vi "Gas Ritter Temperature and Pressure.vi"(0 "Ritter Data":T1, 5 "TC8":dbl, 7 "PSI 1":dbl, 9 "Heise Barometric Pressure (inHG)":dbl, 11 "error in (no error)":errorcluster) -> (4 "Ritter Data Output":T1, 15 "error out":errorcluster)   [LabVIEW 2023]
uses:
  Drivers/Ritter Gas Meter/Type Definitions/Ritter Data.ctl
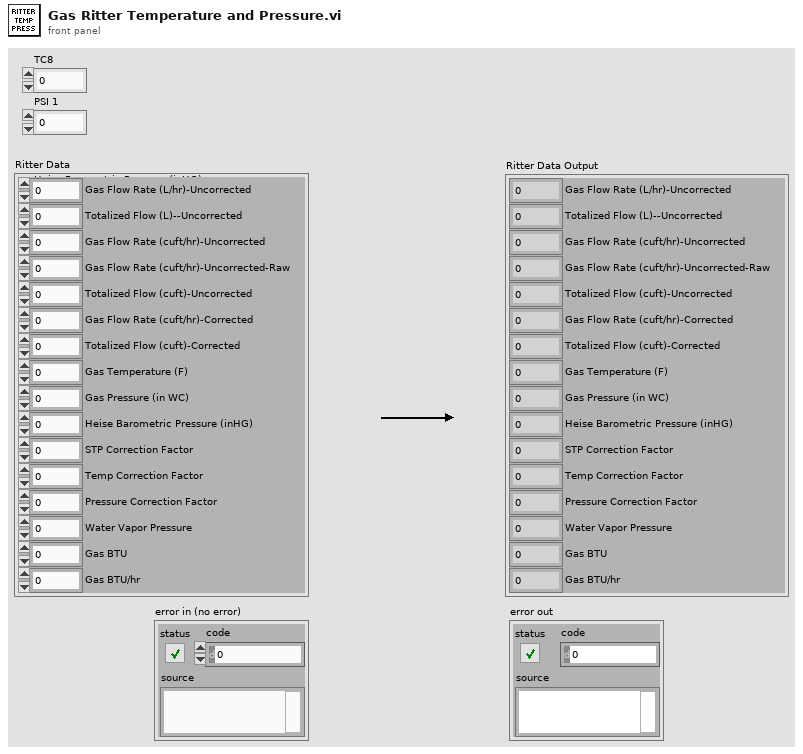
[diagram p1: front panel]
types:
  T1 = typedef "Ritter Data.ctl" = cluster{"Gas Flow Rate (L/hr)-Uncorrected":dbl, "Totalized Flow (L)--Uncorrected":dbl, "Gas Flow Rate (cuft/hr)-Uncorrected":dbl, "Totalized Flow (cuft)-Uncorrected":dbl, "Gas Temperature (F)":dbl, "Gas Pressure (in WC)":dbl, "Heise Barometric Pressure (inHG)":dbl, "STP Correction Factor":dbl, "Temp Correction Factor":dbl, "Pressure Correction Factor":dbl, "Water Vapor Pressure":dbl, "Gas Flow Rate (cuft/hr)-Corrected":dbl, "Totalized Flow (cuft)-Corrected":dbl, "Gas BTU":dbl, "Gas BTU/hr":dbl, "Gas Flow Rate (cuft/hr)-Uncorrected-Raw":dbl}
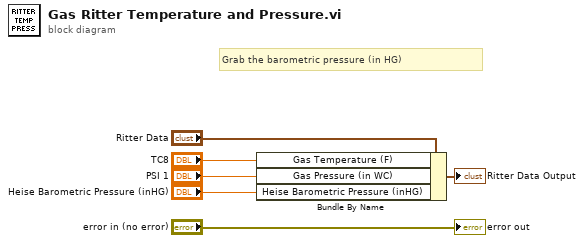
[diagram p0: block diagram]
diagram:
  # "Grab the barometric pressure (in HG)"
  n1 = Bundle By Name(cluster="Ritter Data", "Gas Temperature (F)"="TC8", "Gas Pressure (in WC)"="PSI 1", "Heise Barometric Pressure (inHG)"="Heise Barometric Pressure (inHG)") -> (→"Ritter Data Output":T1)
  "error out" <- "error in (no error)"
